vi "encodeArrayString.vi"(8 "error in (no error)":errorcluster, 11 "String Array":string[](array[string])) -> (0 "error out":errorcluster, 3 "MessagePack":u8[](array[numeric]) format="%.0x")   [LabVIEW 2015, in "MsgPack.lvlib"]
uses:
  MsgPack.lvlib
  encodeString.vi
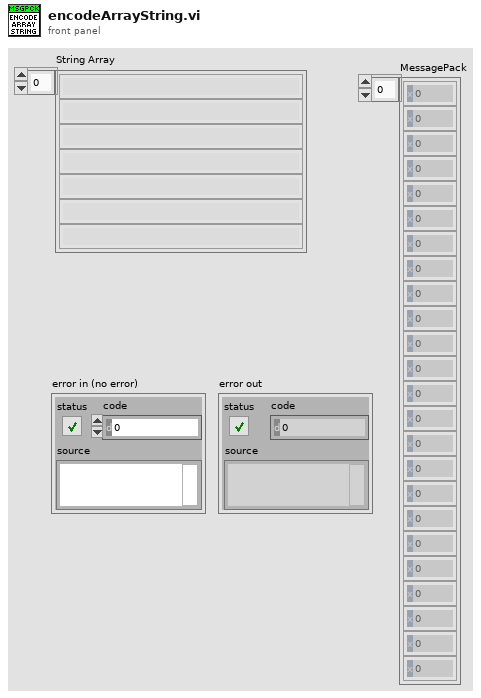
[diagram p1: front panel]
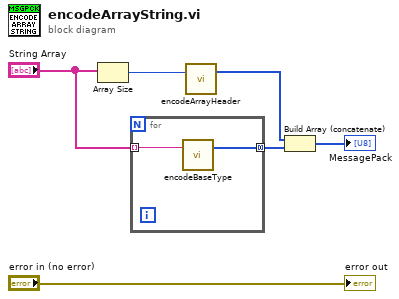
[diagram p0: block diagram]
diagram:
  n1 = Array Size(array="String Array") -> (size(s)=w5:i32)
  n2 = for {
    tunnel: "String Array" -> [w8] mode=indexing
    tunnel: [w7] -> w2 mode=concatenating
    n3 = call-poly "encodeBaseType.vi"("string"=w8) -> ("MessagePack"=w7:u8[])  [unwired: 2 in]
  }
  n4 = call "encodeArrayHeader.vi"("Number of Elements"=w5) -> ("array header"=w4:u8[])  [unwired: 2 in]
  n5 = Build Array (concatenate)(w4, w2) -> (→"MessagePack":u8[])
  "error out" <- "error in (no error)"
